vi "CF Impulse Response.vi"() -> ()   [LabVIEW 2011]
uses:
  <vilib>/imath/engines/lvmath2/RunTimeEngine/ErrorHandling/NIMS_Finalize Error.vi
  <vilib>/imath/engines/lvmath2/RunTimeEngine/Managers/WorkSpace/UID Generator.vi
  <vilib>/imath/engines/lvmath2/RunTimeEngine/Managers/SymbolTable/Clear UID.vi
  <vilib>/imath/engines/lvmath2/RunTimeEngine/NodeEndStatement/NIMS_NodeEndStatement_Output.vi
  <instcachedir>/2/NIMS_NodeEndStatement_Output_53EC0D466D134D7ABD903AC30B43404B.lvgen/NIMS_NodeEndStatement_Output_53EC0D466D134D7ABD903AC30B43404B_003.vi
  <instcachedir>/2/NIMS_NodeEndStatement_Output_53EC0D466D134D7ABD903AC30B43404B.lvgen/NIMS_NodeEndStatement_Output_53EC0D466D134D7ABD903AC30B43404B_001.vi
  <vilib>/imath/engines/lvmath2/RunTimeEngine/RunTimeType/NIMS_RunTimeType_From StrictType (excl LVString).vi
  <instcachedir>/2/NIMS_RunTimeType_From StrictType (excl LVString)_46AE8B54A11948F0BCCEB8091EE7AA4C.lvgen/NIMS_RunTimeType_From StrictType (excl LVString)_46AE8B54A11948F0BCCEB8091EE7AA4C_000.vi
  <vilib>/imath/engines/lvmath2/RunTimeEngine/LocalVariableDefStatement/MC_LocalVariableDefStatement_Display.vi
  <vilib>/imath/engines/lvmath2/RunTimeEngine/Managers/SymbolTable/NIMS_WorkSpace.lvlib
  <vilib>/ptbypt/NI_PtbyPt.lvlib
panel:
  in  "a":dbl(slide) scale=-1.0..1.0
  in  "N":i32(slide) scale=0.0..10.0
  in  "stop":bool
  out "XY Graph":cluster{"Y":dbl[], "Y":dbl[]}[](graph)
  in  "w0":dbl(slide) min=-5.0 max=5.0 step=1.0 scale=-5.0..5.0
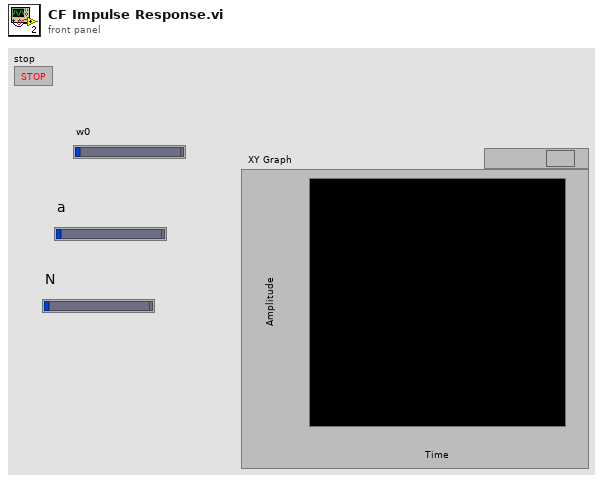
[diagram p1: front panel]
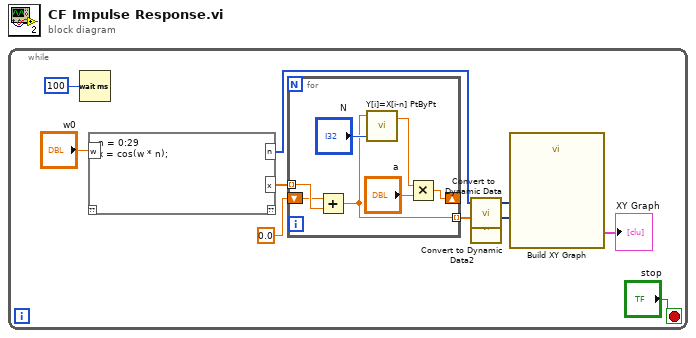
[diagram p0: block diagram]
diagram:
  n1 = while {
    stop <- "stop" stop-if-true
    n2 = Wait (ms)(milliseconds to wait=u32 100) -> ()  [unwired: 1 out]
    n3 = mathscript code="n = 0:29\nx = cos(w * n);"("w"="w0") -> ("x"=w2:dbl[], "n"=w7:i32[])  [unwired: 1 in, 1 out]
    n4 = for {
      tunnel: w2 -> [w57] mode=indexing
      shift-right: [w52] -> _
      shift-left: 0.0 -> [w55]
      tunnel: [w51] -> w1 mode=indexing
      n5 = Add(x=w55, y=w57) -> (x+y=w51:dbl)
      n6 = call <vilib>:"Y[i]=X[i-n] PtByPt.vi"("shifts: n"="N", "x"=w51) -> ("shifted x"=w54:dbl)  [unwired: 2 in, 1 out]
      n7 = Multiply(x=w54, y="a") -> (x*y=w52:dbl)
    }
    n8 = call "Convert to Dynamic Data"("Array"=w7) -> ("Dynamic Data Type"=w6:dynamicdata)  [unwired: 3 in]
    n9 = call "Convert to Dynamic Data2"("Array"=w1) -> ("Dynamic Data Type"=w3:dynamicdata)  [unwired: 3 in]
    n10 = call "Build XY Graph"("Y Input"=w3, "X Input"=w6) -> ("XY Graph"=→"XY Graph":cluster{"Y":dbl[], "Y":dbl[]}[])  [unwired: 3 in, 6 out]
  }
